vi "Legend.vi"(8 "error in (no error)":errorcluster, 10 "Plot labels":string[](array[string]), 11 "ITX Commands in":refnum<class "ITX Commands.lvclass">) -> (0 "error out":errorcluster, 3 "ITX Commands out":refnum<class "ITX Commands.lvclass">)   [LabVIEW 2019, in "ITX Commands.lvclass"]
uses:
  ITX Commands.lvclass
  ITX Commands.lvclass/ITX Commands.ctl
panel:
  out "length":i32
  out "resulting string":string
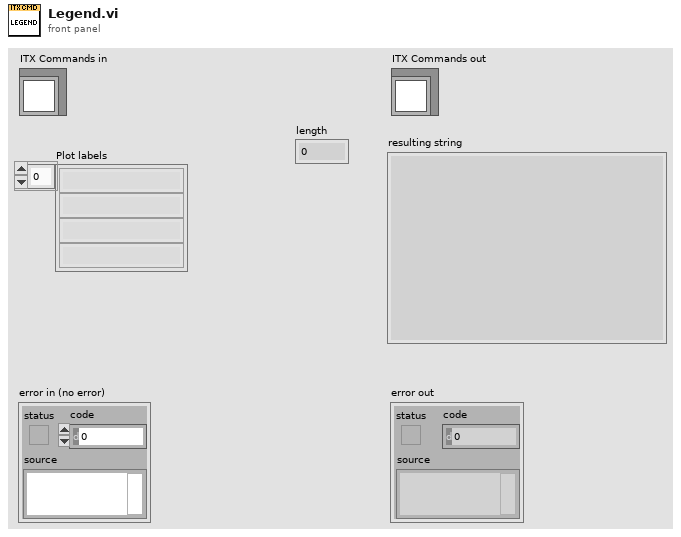
[diagram p1: front panel]
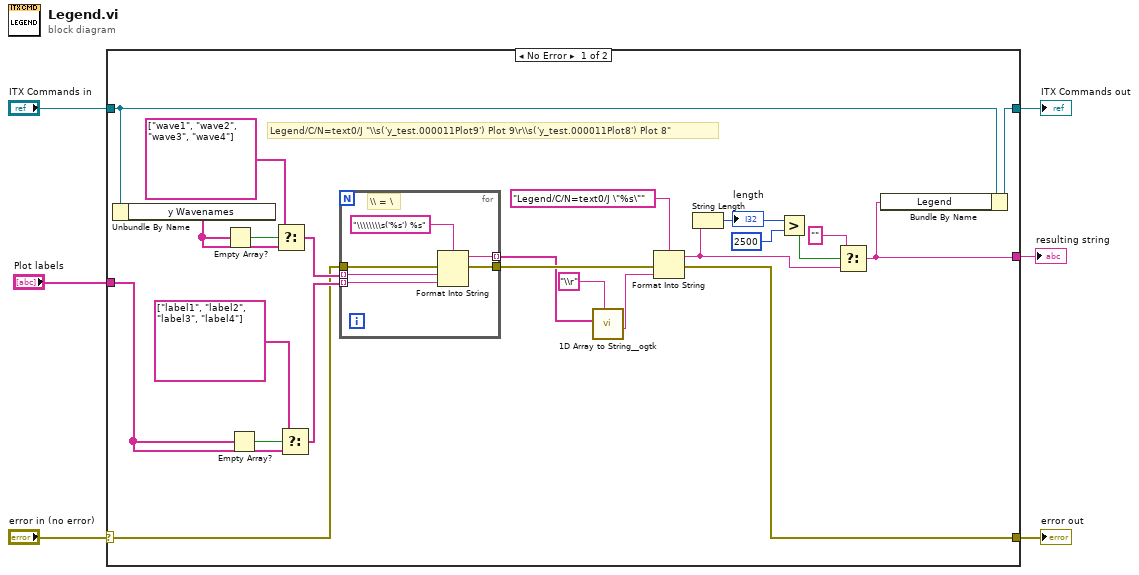
[diagram p0: block diagram]
diagram:
  n1 = case shown="No Error" "error in (no error)" {
    selector: "error in (no error)" -> [w17 w37]
    tunnel: [w23 w37] -> w5
    tunnel: [w29 w36] -> w3
    tunnel: "ITX Commands in" -> [w28 w36]
    tunnel: "Plot labels" -> [w21 _]
    tunnel: [w9 _] -> w1
    frame No Error {
      # "Legend/C/N=text0/J \"\\\\s('y_test.000011Plot9') Plot 9\\r\\\\s('y_test.000011Plot8') Plot 8\""
      n2 = Unbundle By Name(w28) -> ("y Wavenames"=w25:string[])
      n3 = Empty Array?(array=w25) -> (empty?=w26:bool)
      n4 = Empty Array?(array=w21) -> (empty?=w22:bool)
      n5 = Select(t=string[] ["wave1", "wave2", "wave3", "wave4"] ("y Wavenames"), s=w26, f=w25) -> (s? t:f=w24:string[])
      n6 = Select(t=string[] ["label1", "label2", "label3", "label4"] ("y Wavenames"), s=w22, f=w21) -> (s? t:f=w20:string[])
      n7 = for {
        tunnel: w24 -> [w32] mode=indexing
        tunnel: w20 -> [w31] mode=indexing
        tunnel: [w30] -> w14 mode=indexing
        tunnel: w17 -> [w34]
        tunnel: [w35] -> w27
        # "\\\\ = \\"
        n8 = Format Into String(format string="\\\\\\\\s('%s') %s", error in=w34, w32, w31) -> (resulting string=w30:string, error out=w35:errorcluster)  [unwired: 1 in]
      }
      n9 = call <userlib>:"1D Array to String__ogtk.vi"("delimiter (Tab)"="\\r", "Array of Strings"=w14) -> ("delimited string"=w13:string)  [unwired: 9 in]
      n10 = Format Into String(format string="Legend/C/N=text0/J \"%s\"", error in=w27, w13) -> (resulting string=w8:string, error out=w23:errorcluster)  [unwired: 1 in]
      n11 = String Length(string=w8) -> (length=w12:i32)
      "length" <- w12
      n12 = Greater?(x=w12, y=2500) -> (0:w10:bool)
      n13 = Select(t="", s=w10, f=w8) -> (s? t:f=w9:string)
      n14 = Bundle By Name(cluster=w28, "Legend"=w9) -> (w29:refnum<class "ITX Commands.lvclass">)
    }
    frame Error {
    }
  }
  "error out" <- w5
  "ITX Commands out" <- w3
  "resulting string" <- w1
